vi "Send Single Trigger.vi"(8 "error in (no error)":errorcluster, 11 "VNA-CMT S2 S4 in":refnum<class "VNA-CMT S2 S4.lvclass">) -> (0 "error out":errorcluster, 3 "VNA-CMT S2 S4 out":refnum<class "VNA-CMT S2 S4.lvclass">)   [LabVIEW 2020, in "VNA-CMT S2 S4.lvclass"]
doc: "Sent a single trigger for the VNA. It uses the OPC command to wait until completion.\nIt will use (sweeptime * N average * N ports) for the VISA timeout."
uses:
  VNA-CMT S2 S4.lvclass
  C:/Sandbox/RF Bench/Source Code/WiSpry Test Framework/Instruments/Instrument.lvclass
  Instrument.lvclass/Instrument.ctl
  Instrument.lvclass
  <instrlib>/CMT S2 and S4 VNA/CMT S2 and S4 VNA.lvlib
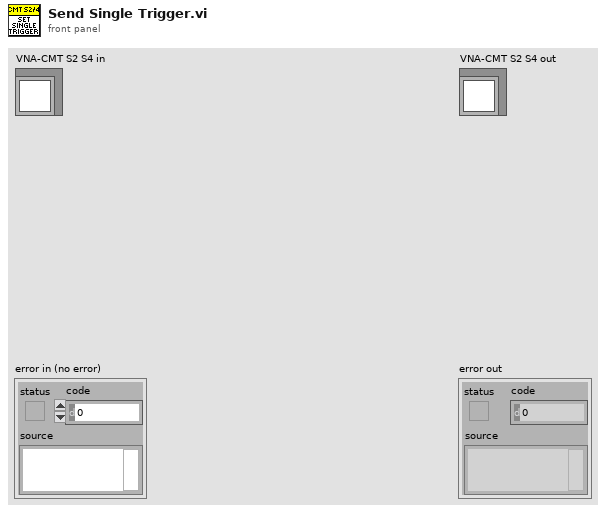
[diagram p1: front panel]
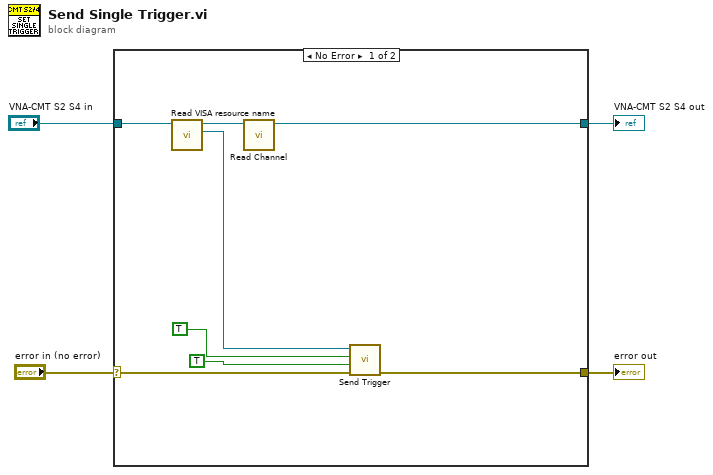
[diagram p0: block diagram]
diagram:
  n1 = case shown="No Error" "error in (no error)" {
    selector: "error in (no error)" -> [w11 w14]
    tunnel: [w8 w14] -> w3
    tunnel: [w5 w13] -> w2
    tunnel: "VNA-CMT S2 S4 in" -> [w12 w13]
    frame No Error {
      n2 = call "Read VISA resource name.vi"("Instrument in"=w12) -> ("VISA resource name"=w9:refnum<visa-resource-name>, "Instrument out"=w6:refnum<class "VNA-CMT S2 S4.lvclass">)  [unwired: 9 in]
      n3 = call-dynamic "Read Channel.vi"("Vector Network Analyzer in"=w6) -> ("Vector Network Analyzer out"=w5:refnum<class "VNA-CMT S2 S4.lvclass">)  [unwired: 9 in, 1 out]
      n4 = call <instrlib>:"Send Trigger.vi"("error in (no error)"=w11, "Wait for OPC (F: Do not Wait)"=TRUE, "Ignore Trigger Source (F: Do not Ignore)"=TRUE, "VISA resource name"=w9) -> ("error out"=w8:errorcluster)  [unwired: 6 in, 1 out]
    }
    frame Error {
    }
  }
  "error out" <- w3
  "VNA-CMT S2 S4 out" <- w2
